vi "preregistration_data_correct.vi"(11 "preregistraion_data":T2) -> (3 "ready":T1(ring))   [LabVIEW 2018]
uses:
  controls/preregistration_data.ctl
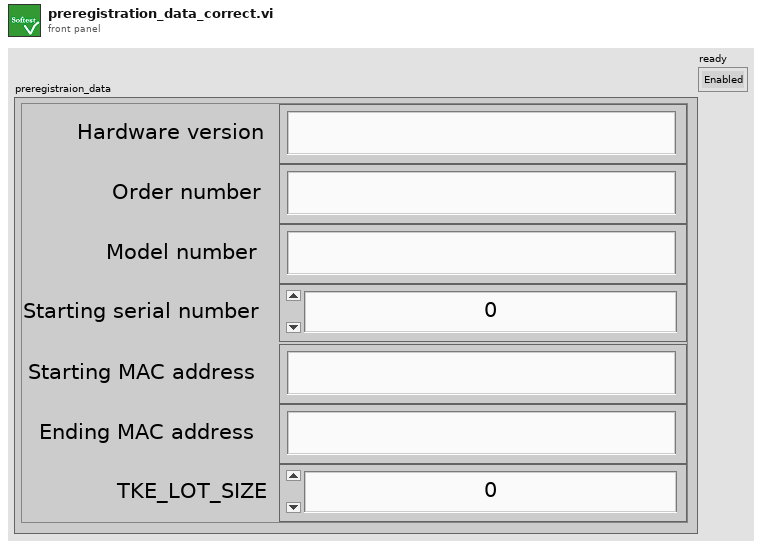
[diagram p1: front panel]
types:
  T1 = enum8{"Enabled", "Disabled", "Disabled and Grayed Out"}
  T2 = typedef "preregistration_data.ctl" = cluster{"Hardware version":string, "Order number":string, "Model number":string, "Starting serial number":i32, "Starting MAC address":string, "Ending MAC address":string, "TKE_LOT_SIZE":i32}
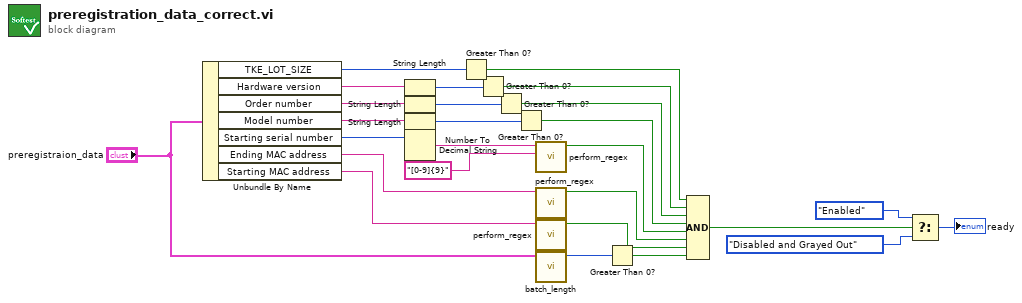
[diagram p0: block diagram]
diagram:
  n1 = Unbundle By Name("preregistraion_data") -> ("TKE_LOT_SIZE"=w16:i32, "Hardware version"=w19:string, "Order number"=w18:string, "Model number"=w17:string, "Starting serial number"=w26:i32, "Ending MAC address"=w23:string, "Starting MAC address"=w22:string)
  n2 = String Length(string=w19) -> (length=w13:i32)
  n3 = String Length(string=w18) -> (length=w14:i32)
  n4 = String Length(string=w17) -> (length=w15:i32)
  n5 = Number To Decimal String(number=w26) -> (decimal integer string=w25:string)  [unwired: 1 in]
  n6 = Greater Than 0?(x=w16) -> (x > 0?=w5:bool)
  n7 = Greater Than 0?(x=w13) -> (x > 0?=w6:bool)
  n8 = Greater Than 0?(x=w14) -> (x > 0?=w7:bool)
  n9 = Greater Than 0?(x=w15) -> (x > 0?=w8:bool)
  n10 = call "perform_regex.vi"("regular expression[MAC address format]"="[0-9]{9}" ("regular expression"), "input string"=w25) -> ("result"=w9:bool)  [unwired: 9 in]
  n11 = call "perform_regex.vi"("input string"=w23) -> ("result"=w10:bool)  [unwired: 10 in]
  n12 = call "perform_regex.vi"("input string"=w22) -> ("result"=w11:bool)  [unwired: 10 in]
  n13 = call "batch_length.vi"("preregistraion_data"="preregistraion_data") -> ("batch_length"=w20:i32)  [unwired: 10 in]
  n14 = Greater Than 0?(x=w20) -> (x > 0?=w12:bool)
  n15 = Compound Arithmetic op=AND(w5, w6, w7, w8, w9, w10, w11, w12) -> (w4:bool)
  n16 = Select(t=T1."Enabled" ("Disabled"), s=w4, f=T1."Disabled and Grayed Out" ("Disabled")) -> (s? t:f=→"ready":T1)
